vi "CRYASIO Out & Init & Start.vi"(8 "Bit Depth":u16=16, 9 "Sampling Rate":u32=44100, 10 "Channel Index":u32, 11 "Device Name":string) -> (2 "bResult":bool, 3 "Asio Opend Channel Index":u32)   [LabVIEW 2013]
uses:
  CRYMisc vis settings global.vi
panel:
  in  "ASIO AMP":dbl=0.1 caption="%" min=0.0 format="%.1f"
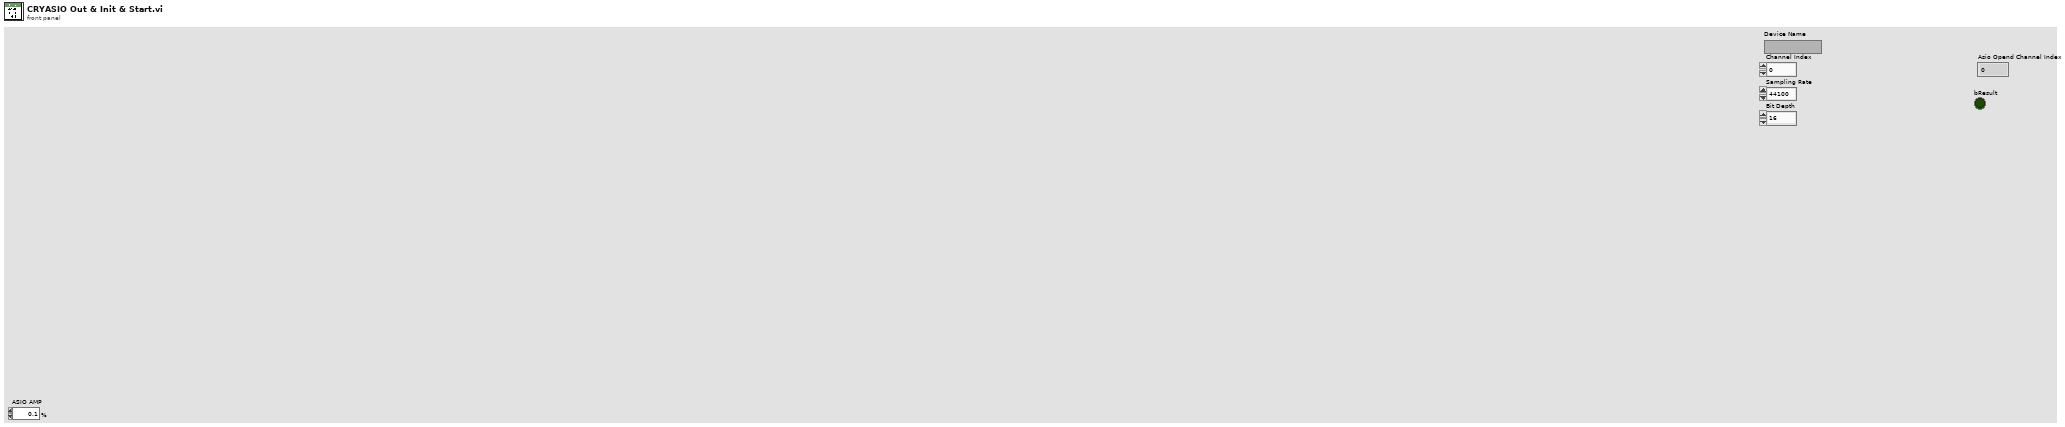
[diagram p1: front panel]
types:
  T1 = cluster{"Chn Name":string, "Count":i16, "Opend Idx":i16}
  T2 = cluster{"Chn Name":string, "Count":i16, "Opend Idx":i16}[]
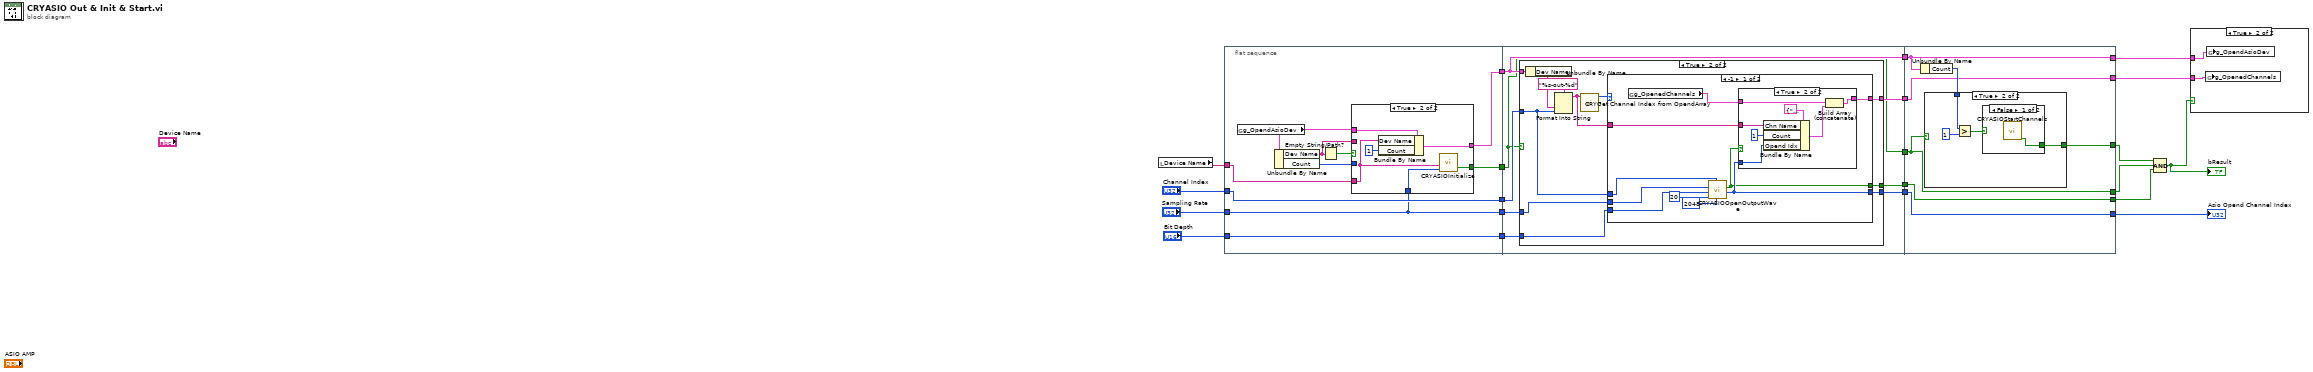
[diagram p0: block diagram]
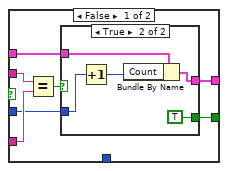
[diagram p3: hidden frame]
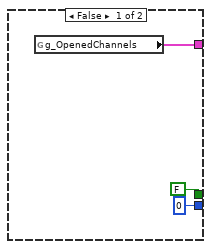
[diagram p5: hidden frame]
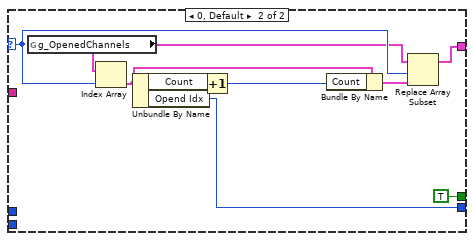
[diagram p7: hidden frame]
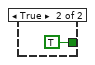
[diagram p9: hidden frame]
diagram:
  n1 = local read "Device Name"() -> (w21:string)
  n2 = flat-sequence {
    tunnel: w21 -> [w29]
    tunnel: "Channel Index" -> [w26]
    tunnel: "Sampling Rate" -> [w25]
    tunnel: [w26] -> w18
    tunnel: [w25] -> w17
    tunnel: "Bit Depth" -> [w24]
    tunnel: [w24] -> w15
    tunnel: [w23] -> w14
    tunnel: [w22] -> w13
    tunnel: w18 -> [w59]
    tunnel: w17 -> [w58]
    tunnel: w15 -> [w57]
    tunnel: w14 -> [w53]
    tunnel: w13 -> [w56]
    tunnel: [w56] -> w12
    tunnel: [w55] -> w11
    tunnel: [w54] -> w10
    tunnel: [w53] -> w9
    tunnel: [w52] -> w5
    tunnel: w12 -> [w106]
    tunnel: w11 -> [w104]
    tunnel: w10 -> [w105]
    tunnel: w9 -> [w103]
    tunnel: [w106] -> w6
    tunnel: [w105] -> w8
    tunnel: [w104] -> w7
    tunnel: [w103] -> w3
    tunnel: w5 -> [w102]
    tunnel: [w102] -> w2
    tunnel: [w101] -> w4
    frame #0 {
      n3 = global read "CRYMisc vis settings global.vi" "g_OpendAsioDev"() -> (w30:cluster{"Dev Name":string, "Count":i16})
      n4 = Unbundle By Name(w30) -> ("Dev Name"=w28:string, "Count"=w27:i16)
      n5 = Empty String/Path?(string/path=w28) -> (empty?=w31:bool)
      n6 = case shown="True" w31 {
        tunnel: w30 -> [w35 w51]
        tunnel: w29 -> [w37 w49]
        tunnel: w25 -> [_ w48]
        tunnel: w28 -> [w38 _]
        tunnel: w27 -> [w34 _]
        tunnel: [w33 w47] -> w22
        tunnel: [w32 w46] -> w23
        frame False {
          n7 = Equal?(x=w38, y=w37) -> (x = y?=w36:bool)
          n8 = case shown="True" w36 {
            selector: w36 -> [w39 _]
            tunnel: w35 -> [w40 w45]
            tunnel: w34 -> [_ w44]
            tunnel: [w40 w42] -> w33
            tunnel: [w39 TRUE] -> w32
            frame False {
            }
            frame True {
              n9 = Increment(x=w44) -> (x+1=w43:i16)
              n10 = Bundle By Name(cluster=w45, "Count"=w43) -> (w42:cluster{"Dev Name":string, "Count":i16})
            }
          }
        }
        frame True, Default {
          n11 = Bundle By Name(cluster=w51, "Dev Name"=w49, "Count"=i16 1) -> (w47:cluster{"Dev Name":string, "Count":i16})
          n12 = call "CRYASIOInitialize.vi"("Sampling Rate"=w48, "Driver Name"=w49) -> ("bResult"=w46:bool)  [unwired: 8 in, 1 out]
        }
      }
    }
    frame #1 {
      n13 = case shown="True" w53 {
        tunnel: w56 -> [_ w73]
        tunnel: w59 -> [_ w68]
        tunnel: w58 -> [_ w67]
        tunnel: w57 -> [_ w66]
        tunnel: [w62 w65] -> w55
        tunnel: [u32 0 ("Limit") w64] -> w54
        tunnel: [FALSE ("bResult") w63] -> w52
        frame False {
          n14 = global read "CRYMisc vis settings global.vi" "g_OpenedChannels"() -> (w62:T2)
        }
        frame True {
          n15 = Unbundle By Name(w73) -> ("Dev Name"=w72:string)
          n16 = Format Into String(format string="%s-out-%d", w72, w68) -> (resulting string=w69:string)  [unwired: 2 in, 1 out]
          n17 = call "CRYGet Channel Index from OpendArray.vi"("Channel Name"=w69) -> ("index of Channel"=w70:i32)  [unwired: 10 in]
          n18 = case shown="-1" w70 {
            selector: w70 -> [_ w97]
            tunnel: w69 -> [w83 _]
            tunnel: [w81 w94] -> w65
            tunnel: w68 -> [w80 _]
            tunnel: w67 -> [w79 _]
            tunnel: w66 -> [w78 _]
            tunnel: [w75 w93] -> w64
            tunnel: [w74 TRUE ("bResult")] -> w63
            frame -1 {
              n19 = global read "CRYMisc vis settings global.vi" "g_OpenedChannels"() -> (w82:T2)
              n20 = call "CRYASIOOpenOutputWave.vi"("Buff Length"=u32 2048 ("Wave Length"), "Channel Index"=w80, "Buff Count"=u32 20 ("Unknown"), "Bit Depth"=w78, "Sampling Rate"=w79) -> ("OCI"=w75:u32, "bResult"=w74:bool)  [unwired: 3 in, 1 out]
              n21 = case shown="True" w74 {
                tunnel: w83 -> [_ w91]
                tunnel: w82 -> [w84 w89]
                tunnel: [w84 w87] -> w81
                tunnel: w75 -> [_ w85]
                frame False {
                }
                frame True {
                  n22 = Bundle By Name(cluster=T1 {"Chn Name"="", "Count"=0, "Opend Idx"=0} ("element"), "Chn Name"=w91, "Count"=i16 1, "Opend Idx"=w85) -> (w88:T1)
                  n23 = Build Array (concatenate)(w89, w88) -> (w87:T2)
                }
              }
            }
            frame 0, Default {
              n24 = global read "CRYMisc vis settings global.vi" "g_OpenedChannels"() -> (w96:T2)
              n25 = Index Array(array=w96, index=w97) -> (element=w100:T1)
              n26 = Unbundle By Name(w100) -> ("Count"=w98:i16, "Opend Idx"=w93:i16)
              n27 = Increment(x=w98) -> (x+1=w99:i16)
              n28 = Bundle By Name(cluster=w100, "Count"=w99) -> (w95:T1)
              n29 = Replace Array Subset(array=w96, new element=w95, index=w97) -> (w94:T2)
            }
          }
        }
      }
    }
    frame #2 {
      n30 = Unbundle By Name(w106) -> ("Count"=w107:i16)
      n31 = case shown="True" w103 {
        selector: w103 -> [w108 _]
        tunnel: w107 -> [_ w112]
        tunnel: [w108 w109] -> w101
        frame False {
        }
        frame True {
          n32 = Greater?(x=w112, y=i16 1) -> (0:w110:bool)
          n33 = case shown="False" w110 {
            tunnel: [w113 TRUE ("bResult")] -> w109
            frame False {
              n34 = call "CRYASIOStartChannels.vi"() -> ("bResult"=w113:bool)  [unwired: 10 in, 1 out]
            }
            frame True {
            }
          }
        }
      }
    }
  }
  n35 = Compound Arithmetic op=AND(w4, w3, w2) -> (w1:bool)
  "bResult" <- w1
  n36 = case shown="True" w1 {
    tunnel: w7 -> [_ w116]
    tunnel: w6 -> [_ w115]
    frame False {
    }
    frame True {
      n37 = global write "CRYMisc vis settings global.vi" "g_OpenedChannels"(w116) -> ()
      n38 = global write "CRYMisc vis settings global.vi" "g_OpendAsioDev"(w115) -> ()
    }
  }
  "Asio Opend Channel Index" <- w8
